vi "Grove Thumb Joystick.vi"() -> ()   [LabVIEW 2020, in "CTI-Scratchpad.lvlib"]
uses:
  CTI-Scratchpad.lvlib
  CTI/Error Reporting.ctl
  CTI/Identity.ctl
  CTI/ADC Number.ctl
  CTI/Session/Session.lvclass
  CTI/CTI.lvlib
  CTI/VisaComms/VisaComms.lvclass
panel:
  out "XY Graph":cluster{"X":u16, "Y":i16}[](graph)
  out "Identity":T1
  in  "GroveConnector":enum16{"A0", "A1", "A2"}(ring)=enum."A1"
  in  "Error Checking (Full)":T2
  in  "Speed(ms)":i32(slide)=12 scale=1000.0..1.0
  in  "stop":bool
  in  "Port":refnum<visa-resource-name>="TCPIP::10.190.177.58::5555::SOCKET"
  # "https://wiki.seeedstudio.com/Grove-Thumb_Joystick/"
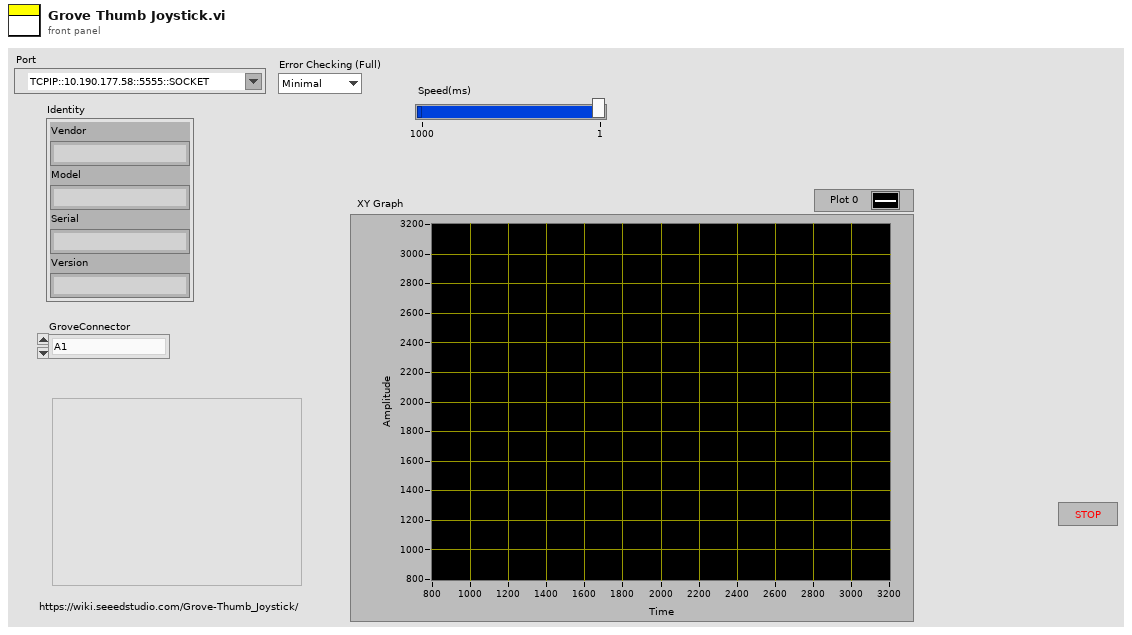
[diagram p1: front panel]
types:
  T1 = typedef "CTI.lvlib/Identity.ctl" = cluster{"Vendor":string, "Model":string, "Serial":string, "Version":string}
  T2 = typedef "CTI.lvlib/Error Reporting.ctl" = enum16{"Minimal", "Moderate", "Full"}
  T3 = typedef "CTI.lvlib/ADC Number.ctl" = i8
  T4 = typedef "CTI.lvlib/Raw ADC.ctl" = u16
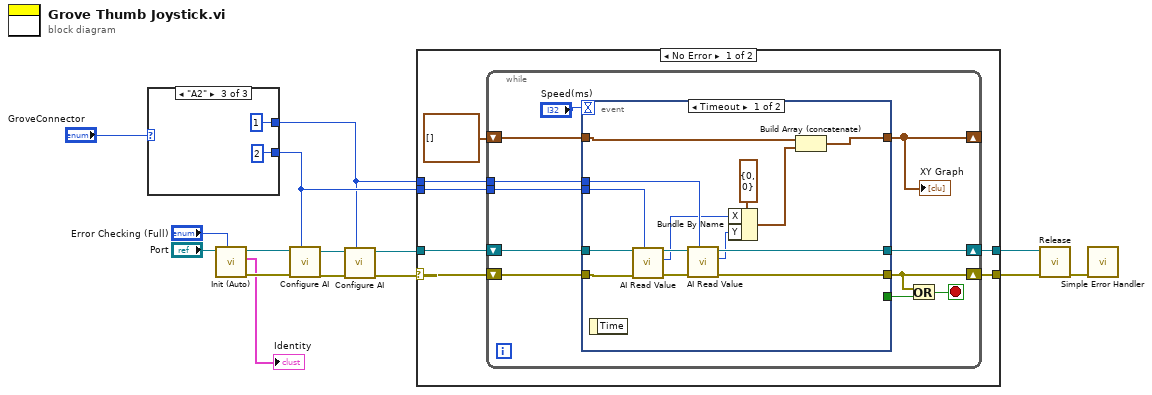
[diagram p0: block diagram]
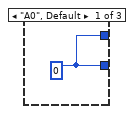
[diagram p2: hidden frame]
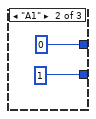
[diagram p3: hidden frame]
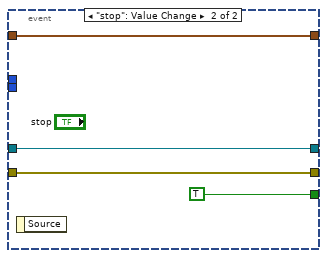
[diagram p4: hidden frame]
diagram:
  n1 = case shown="\"A2\"" "GroveConnector" {
    tunnel: [w16 T3 1 T3 2] -> w6
    tunnel: [w16 T3 0 T3 1] -> w3
    frame "A0", Default {
      w16 = T3 0
    }
    frame "A1" {
    }
    frame "A2" {
    }
  }
  n2 = call "Init (Auto).vi"("Error Checking (Full)"="Error Checking (Full)", "VISA resource name"="Port") -> ("error out"=w13:errorcluster, "Identity"=→"Identity":T1, "Session"=w14:refnum<class "Session.lvclass">)  [unwired: 7 in]
  n3 = call "Configure AI.vi"("ADC #"=w6, "error in (no error)"=w13, "Session in"=w14) -> ("error out"=w5:errorcluster, "Session out"=w4:refnum<class "Session.lvclass">)  [unwired: 7 in]
  n4 = call "Configure AI.vi"("ADC #"=w3, "error in (no error)"=w5, "Session in"=w4) -> ("error out"=w2:errorcluster, "Session out"=w1:refnum<class "Session.lvclass">)  [unwired: 7 in]
  n5 = case shown="No Error" w2 {
    selector: w2 -> [w25 w58]
    tunnel: w1 -> [w26 w57]
    tunnel: w6 -> [w27 _]
    tunnel: [w23 w58] -> w11
    tunnel: [w24 w57] -> w12
    tunnel: w3 -> [w22 _]
    frame No Error {
      n6 = while {
        tunnel: w27 -> [w37]
        shift-right: [w34] -> w24
        shift-left: w26 -> [w36]
        shift-right: [w33] -> w23
        shift-left: w25 -> [w35]
        tunnel: w22 -> [w28]
        shift-right: [w29] -> _
        shift-left: cluster{"X":u16, "Y":i16}[] [] ("XY Graph") -> [w30]
        stop <- w31 stop-if-true
        n7 = event shown="[0] Timeout" {
          selector: _ -> [_ _]
          dyn-events: _ -> [_ _]
          timeout: "Speed(ms)" -> [_ _]
          tunnel: w37 -> [w46 _]
          tunnel: w36 -> [w48 w54]
          tunnel: w35 -> [w47 w55]
          tunnel: [w52 w54] -> w34
          tunnel: [w51 w55] -> w33
          tunnel: [_ TRUE] -> w32
          tunnel: w30 -> [w41 w53]
          tunnel: [w39 w53] -> w29
          tunnel: w28 -> [w45 _]
          event Timeout {
            n8 = event-data() -> ()  [unwired: 1 in, 1 out]
            n9 = call "AI Read Value.vi"("ADC #"=w46, "error in (no error)"=w47, "Session in"=w48) -> ("error out"=w50:errorcluster, "Value"=w43:T4, "Session out"=w49:refnum<class "Session.lvclass">)  [unwired: 6 in]
            n10 = call "AI Read Value.vi"("ADC #"=w45, "error in (no error)"=w50, "Session in"=w49) -> ("error out"=w51:errorcluster, "Value"=w42:T4, "Session out"=w52:refnum<class "Session.lvclass">)  [unwired: 6 in]
            n11 = Bundle By Name(cluster=cluster{"X":u16, "Y":i16} {"X"=0, "Y"=0}, "X"=w43, "Y"=w42) -> (w40:cluster{"X":u16, "Y":i16})
            n12 = Build Array (concatenate)(w41, w40) -> (w39:cluster{"X":u16, "Y":i16}[])
          }
          event "stop": Value Change {
            n13 = event-data() -> ()  [unwired: 1 in, 1 out]
          }
        }
        "XY Graph" <- w29
        n14 = Or(x=w33, y=w32) -> (x .or. y?=w31:bool)
      }
    }
    frame Error {
    }
  }
  n15 = call-dynamic "Release.vi"("error in (no error)"=w11, "Session in"=w12) -> ("error out"=w10:errorcluster)  [unwired: 9 in]
  n16 = call <vilib>:"Simple Error Handler.vi"("error in (no error)"=w10) -> ()  [unwired: 4 in, 5 out]
